vi "9_Meas_Tf.vi"(0 "file path (IN)":path, 1 "ICE":dbl, 5 "Project #":string, 7 "Request #":string, 9 "TEST #":string, 11 "error in (no error)":errorcluster) -> (4 "file path (OUT)":path, 6 "Tf (ns)":dbl, 8 "DONE Tf":bool, 10 "OFF Region":waveform(dbl)[](graph) caption="Tf (ns)", 15 "error out":errorcluster)   [LabVIEW 2020]
uses:
  <vilib>/Waveform/WDTOps.llb/WDT Waveform Duration DBL.vi
  <vilib>/Waveform/WDTOps.llb/WDT Get Waveform Subset DBL.vi
  <vilib>/measure/mascope.llb/Transition Measurements 1 chan.vi
  <vilib>/measure/NI_MAPro.lvlib
panel:
  in  "Decision ?":bool
  in  "Cursor b : Channel 1 \nfall edge tolerance":dbl=0.1
  in  "Cursor b : Channel 1 \nfall edge number":i32=1 min=1
  in  "Cursor a : Channel 1 \nfall edge tolerance":dbl=0.1
  in  "Cursor a : Channel 1 \nfall edge number":i32=1 min=1
  out "Cursor a : Channel 1":dbl
  out "Cursor b : Channel 1":dbl
  out "10% Ice":dbl
  out "90% Ice":dbl
  out "measurement info (CH1 Cursor a)":T1 {"ref levels"."ref units" items=["absolute", "relative"]; "ref levels"."high ref level" format="%.2p"; "ref levels"."low ref level" format="%.2p"; "ref levels"."mid ref level" format="%.2p"; "end time" format="%.6e"; "start time" format="%.6e"}
  out "measurement info (CH1 Cursor b)":T1 {"ref levels"."ref units" items=["absolute", "relative"]; "ref levels"."high ref level" format="%.2p"; "ref levels"."low ref level" format="%.2p"; "ref levels"."mid ref level" format="%.2p"; "end time" format="%.6e"; "start time" format="%.6e"}
  in  "reference  levels (CH1 2nd Cursor)":T2={"high ref level"=90.0, "mid ref level"=50.0, "low ref level"=10.0, "ref units"=1} {"ref units" items=["absolute", "percent"]; "high ref level" format="%0.2f"; "low ref level" format="%0.2f"; "mid ref level" format="%0.2f"}
  in  "reference  levels (CH1 1st Cursor)":T2={"high ref level"=90.0, "mid ref level"=50.0, "low ref level"=10.0, "ref units"=1} {"ref units" items=["absolute", "percent"]; "high ref level" format="%0.2f"; "low ref level" format="%0.2f"; "mid ref level" format="%0.2f"}
  out "Waveform Graph":waveform(dbl)[](graph)
  # "From 90% Ice to 10% Ice"
  # "Default = 1"
  # "Default = 1"
  # "Default = 0.1"
  # "Default = 0.1"
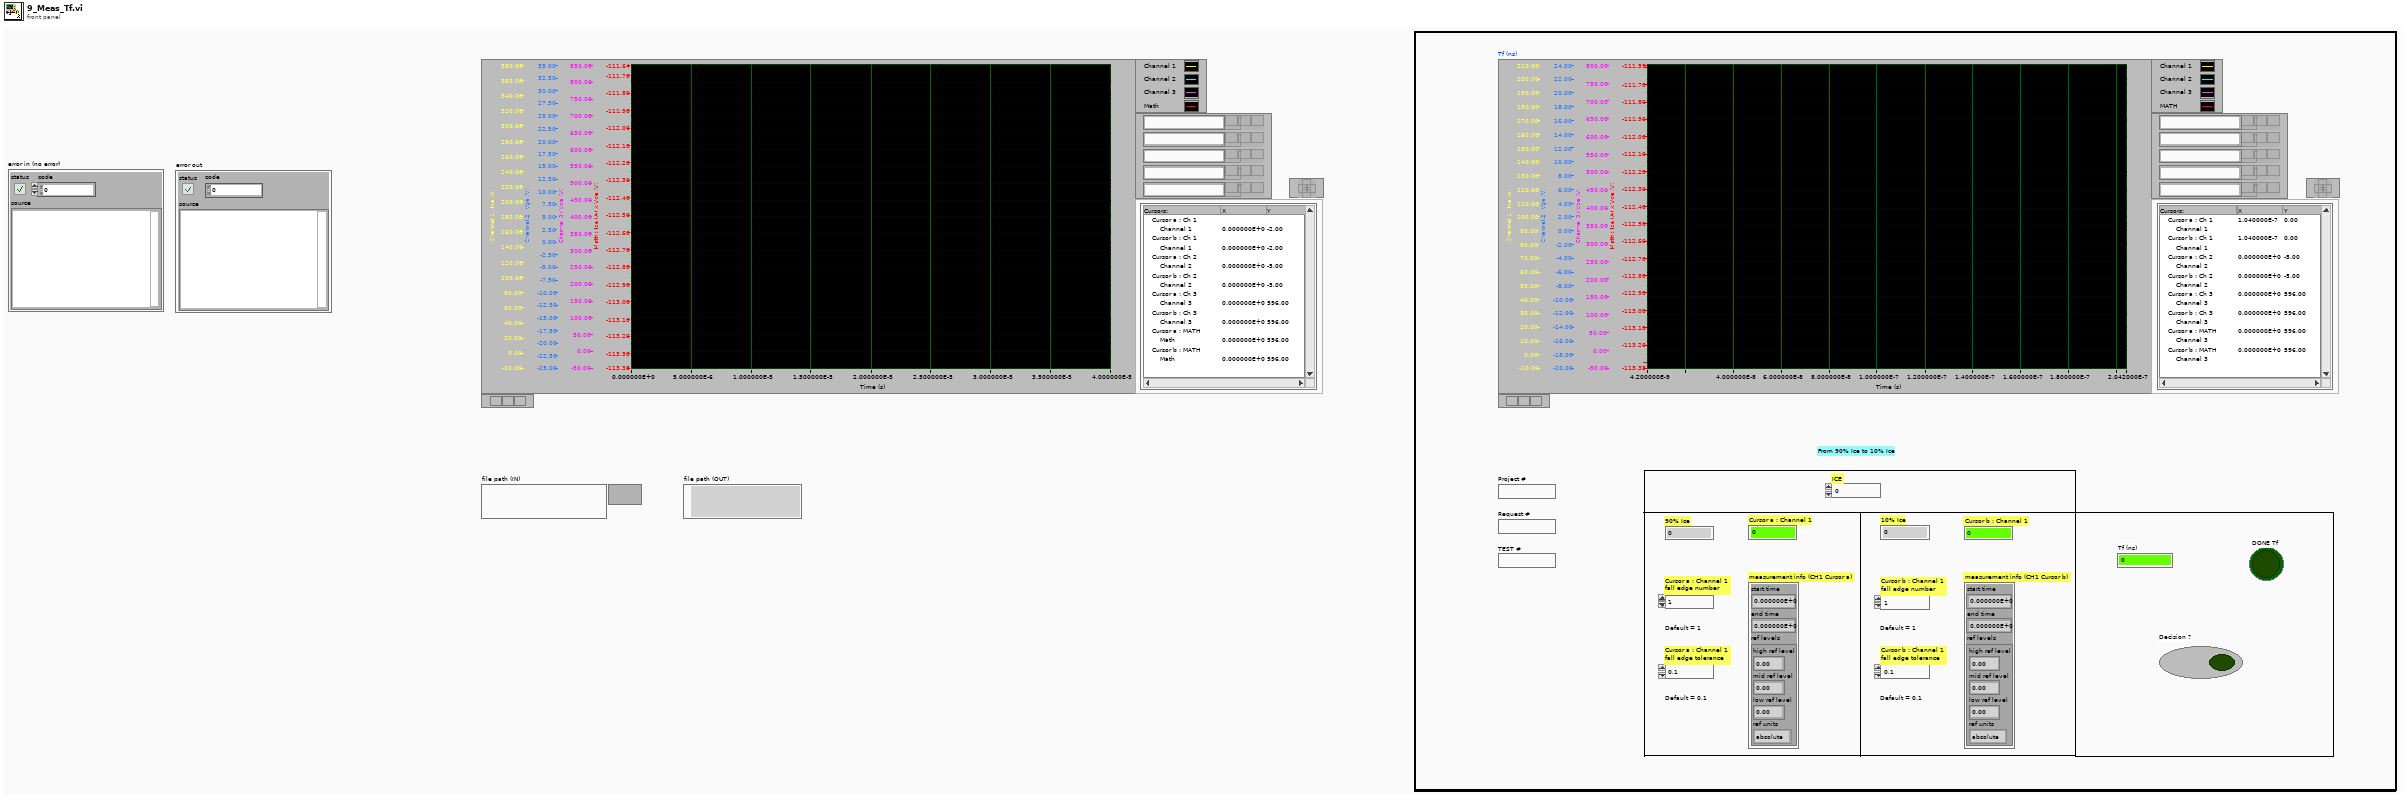
[diagram p1: front panel]
types:
  T1 = cluster{"start time":dbl, "end time":dbl, "ref levels":cluster{"high ref level":dbl, "mid ref level":dbl, "low ref level":dbl, "ref units":u16}}
  T2 = cluster{"high ref level":dbl, "mid ref level":dbl, "low ref level":dbl, "ref units":u16}
  T3 = enum32{"Invalid", "Standard", "Closed", "Hidden", "Minimized", "Maximized"}
  T4 = typedef "imagedata.ctl" = cluster{"image type":i32, "image depth":i32, "image":u8[], "mask":u8[], "colors":u32[], "Rectangle":cluster{"left":i16, "top":i16, "right":i16, "bottom":i16}}
diagram:
  w11 = 0.0 ("Cursor a : Channel 1")
  w13 = errorcluster {"status"=FALSE, "code"=0, "source"=""} ("error out")
  w12 = FALSE ("DONE Tdon")
  w14 = waveform(dbl)[] [] ("Waveform Graph")
  n1 = local write "Cursor a : Channel 1 \nfall edge tolerance"(0.1 ("Cursor a : Channel 1 \nfall edge tolerance")) -> ()
  n2 = local write "Cursor a : Channel 1 \nfall edge number"(1 ("Cursor a : Channel 1 \nfall edge number")) -> ()
  n3 = local write "Cursor b : Channel 1 \nfall edge tolerance"(0.1 ("Cursor b : Channel 1 \nfall edge tolerance")) -> ()
  n4 = local write "Cursor b : Channel 1 \nfall edge number"(1 ("Cursor b : Channel 1 \nfall edge number")) -> ()
  n5 = local write "error out"(w13) -> ()
  n6 = local write "error in (no error)"(w13) -> ()
  n7 = local write "Cursor a : Channel 1"(w11) -> ()
  n8 = local write "Cursor b : Channel 1"(w11) -> ()
  n9 = local write "DONE Tf"(w12) -> ()
  n10 = local write "Waveform Graph"(w14) -> ()
  n11 = local write "OFF Region"(w14) -> ()
  n12 = local write "Decision ?"(w12) -> ()
  n13 = local write "Tf (ns)"(w11) -> ()
  n14 = flat-sequence {
    tunnel: ["file path (IN)"] -> w6
    tunnel: [w15] -> w5
    tunnel: [w26] -> w10
    tunnel: [w25] -> w8
    tunnel: w6 -> [w24]
    tunnel: w5 -> [w23]
    tunnel: w10 -> [w247]
    tunnel: [w246] -> w9
    tunnel: w8 -> [w246]
    tunnel: [w245] -> w7
    tunnel: w9 -> [w261]
    tunnel: w7 -> [w260]
    frame #0 {
      n15 = control-ref of="This VI"() -> (w21:refnum<vi>)
      n16 = invoke class="VI" method="FP.Open"(reference=w21, error in="error in (no error)", "Activate"=TRUE ("Activate?"), "State"=T3."Maximized") -> (error out=w22:errorcluster)  [unwired: 1 in, 4 out]
      n17 = property class="VI"(reference=w21, error in=w22, "Front Panel.Closeable"=TRUE ("Front Panel Window:Closeable")) -> (error out=w15:errorcluster)  [unwired: 1 out]
    }
    frame #1 {
      n18 = while {
        shift-right: [w32] -> w26
        shift-left: w23 -> [w31]
        tunnel: [w28] -> w25
        tunnel: w24 -> [w27]
        stop <- w33 stop-if-true
        n19 = flat-sequence {
          tunnel: w31 -> [w62]
          tunnel: [w62] -> w30
          tunnel: [w57] -> w29
          tunnel: w27 -> [w57]
          tunnel: [w78] -> w50
          tunnel: [w77] -> w49
          tunnel: [w67] -> w48
          tunnel: w30 -> [w155]
          tunnel: w29 -> [w149]
          tunnel: w50 -> [w184]
          tunnel: w49 -> [w198]
          tunnel: [w178] -> w47
          tunnel: w48 -> [w191]
          tunnel: [w191] -> w46
          tunnel: [w177] -> w45
          tunnel: [w176] -> w44
          tunnel: [w175] -> w43
          tunnel: [w174] -> w42
          tunnel: w47 -> [w226]
          tunnel: [w225] -> w41
          tunnel: w46 -> [w227]
          tunnel: [w227] -> w40
          tunnel: w45 -> [_]
          tunnel: w44 -> [_]
          tunnel: w43 -> [w219]
          tunnel: [w219] -> w39
          tunnel: w42 -> [w220]
          tunnel: [w220] -> w38
          tunnel: w41 -> [w228]
          tunnel: w40 -> [w234]
          tunnel: [w234] -> w37
          tunnel: w39 -> [w232]
          tunnel: w38 -> [w231]
          tunnel: [w228] -> w36
          tunnel: w37 -> [w239]
          tunnel: w36 -> [w241]
          tunnel: [w240] -> w35
          tunnel: [w239] -> w28
          frame #0 {
            w60 = 0.0 ("Cursor a : Channel 1")
            w59 = FALSE ("DONE Tdon")
            w58 = waveform(dbl)[] [] ("Waveform Graph")
            n20 = Wait (ms)(milliseconds to wait=u32 200) -> ()  [unwired: 1 out]
            n21 = local write "Cursor a : Channel 1"(w60) -> ()
            n22 = local write "Cursor b : Channel 1"(w60) -> ()
            n23 = local write "DONE Tf"(w59) -> ()
            n24 = local write "Waveform Graph"(w58) -> ()
            n25 = local write "OFF Region"(w58) -> ()
            n26 = local write "Decision ?"(w59) -> ()
            n27 = local write "Tf (ns)"(w60) -> ()
          }
          frame #1 {
            w63 = 0.0 ("start samples/time")
            w130 = u16 1 items=["Samples", "Relative Time"] ("start/duration format")
            w141 = u16 1 items=["Samples", "Relative Time"] ("start/duration format")
            w142 = u16 1 items=["Samples", "Relative Time"] ("start/duration format")
            # "Channel 1"
            # "Channel 3"
            # "Channel 2"
            # "dt"
            # "Ch2"
            # "Ch1"
            n28 = call "3_ReadDatatoWaveform.vi"("error in (no error)"=w155, "file path (IN)"=w149) -> ("error out"=w123:errorcluster, "Waveform Graph"=→"Waveform Graph":waveform(dbl)[], "file path (OUT)"=w67:path, "dt"=w150:dbl, "Ch 2 Data"=w147:dbl[], "Ch 3 Data"=w151:dbl[], "Ch 1 Data"=w148:dbl[])  [unwired: 3 in]
            n29 = To Time Stamp(1:0.0 ("number")) -> (0:w152:timestamp)
            n30 = disable-structure shown="Enabled" {
              disable-tunnel: w152 -> [w159 _]
              disable-tunnel: w150 -> [w158 _]
              disable-tunnel: w148 -> [w157 _]
              disable-tunnel: [w156 _] -> w129
              frame Enabled {
                # "Channel 1"
                n31 = Bundle By Name("Y"=w157, "dt"=w158, "t0"=w159) -> (w156:waveform(dbl))  [unwired: 1 in]
              }
              frame Disabled {
              }
            }
            n32 = disable-structure shown="Enabled" {
              disable-tunnel: w152 -> [w163 _]
              disable-tunnel: w150 -> [w162 _]
              disable-tunnel: w147 -> [w161 _]
              disable-tunnel: [w160 _] -> w128
              frame Enabled {
                # "Channel 2"
                n33 = Bundle By Name("Y"=w161, "dt"=w162, "t0"=w163) -> (w160:waveform(dbl))  [unwired: 1 in]
              }
              frame Disabled {
              }
            }
            n34 = disable-structure shown="Enabled" {
              disable-tunnel: w152 -> [w167 _]
              disable-tunnel: w150 -> [w166 _]
              disable-tunnel: w151 -> [w165 _]
              disable-tunnel: [w164 _] -> w127
              frame Enabled {
                # "Channel 3"
                n35 = Bundle By Name("Y"=w165, "dt"=w166, "t0"=w167) -> (w164:waveform(dbl))  [unwired: 1 in]
              }
              frame Disabled {
              }
            }
            n36 = call-poly <vilib>:"Waveform Duration.vi"("error in (no error)"=w123, "waveform in"=w127) -> ("error out"=w135:errorcluster, "duration"=w132:dbl, "waveform out"=w134:waveform(dbl))  [unwired: 7 in]
            n37 = call-poly <vilib>:"Waveform Duration.vi"("error in (no error)"=w123, "waveform in"=w128) -> ("error out"=w136:errorcluster, "duration"=w139:dbl, "waveform out"=w137:waveform(dbl))  [unwired: 7 in]
            n38 = call-poly <vilib>:"Waveform Duration.vi"("error in (no error)"=w123, "waveform in"=w129) -> ("error out"=w146:errorcluster, "duration"=w143:dbl, "waveform out"=w145:waveform(dbl))  [unwired: 7 in]
            n39 = Divide(x=w132, y=2.0) -> (x/y=w131:dbl)
            n40 = Divide(x=w139, y=2.0) -> (x/y=w140:dbl)
            n41 = Divide(x=w143, y=2.0) -> (x/y=w124:dbl)
            n42 = call-poly <vilib>:"Get Waveform Subset.vi"("start/duration format"=w130, "error in (no error)"=w135, "duration"=w131, "start samples/time"=w63, "waveform in"=w134) -> ("error out"=w120:errorcluster, "waveform out"=w126:waveform(dbl))  [unwired: 1 in, 2 out]
            n43 = call-poly <vilib>:"Get Waveform Subset.vi"("start/duration format"=w141, "error in (no error)"=w136, "duration"=w140, "start samples/time"=w63, "waveform in"=w137) -> ("error out"=w121:errorcluster, "waveform out"=w79:waveform(dbl))  [unwired: 1 in, 2 out]
            n44 = call-poly <vilib>:"Get Waveform Subset.vi"("start/duration format"=w142, "error in (no error)"=w146, "duration"=w124, "start samples/time"=w63, "waveform in"=w145) -> ("error out"=w122:errorcluster, "waveform out"=w78:waveform(dbl))  [unwired: 1 in, 2 out]
            n45 = Build Array(w78, w79, w126) -> (→"OFF Region":waveform(dbl)[])
            n46 = Merge Errors(w122, w121, w120) -> (w75:errorcluster)
            n47 = property on="OFF Region" class="WFGraph (strict)"(error in=w75) -> (error out=w74:errorcluster, "Width"=w73:u32)  [unwired: 1 in, 1 out]
            n48 = property on="OFF Region" class="WFGraph (strict)"(error in=w74, "Caption.Justify"=enum16{"Left", "Center", "Right"}."Left" ("Caption.Justification"), "Caption.Width"=w73, "Caption.FontBold"=TRUE ("Caption.Font:Bold"), "Caption.FontColor"=u32 16860 ("Caption.Font:Color"), "Caption.FontSize"=u32 24 ("Caption.Font:Size"), "Caption.Text"="Tf (ns)") -> (error out=w69:errorcluster)  [unwired: 1 in, 1 out]
            n49 = property on="OFF Region" class="WFGraph (strict)"(error in=w69, "XScale.Offset"=w63) -> (error out=w103:errorcluster)  [unwired: 1 in, 1 out]
            n50 = property on="OFF Region" class="WFGraph (strict)"(error in=w103, "Active Cursor"=u32 0, "Cursor.Cursor X"=0.0 ("Cursor.Cursor Position:Cursor X"), "Cursor.Cursor Y"=0.0 ("Cursor.Cursor Position:Cursor Y"), "Cursor.Visible"=FALSE) -> (error out=w102:errorcluster)  [unwired: 1 in, 1 out]
            n51 = property on="OFF Region" class="WFGraph (strict)"(error in=w102, "Active Cursor"=u32 1, "Cursor.Cursor X"=0.0 ("Cursor.Cursor Position:Cursor X"), "Cursor.Cursor Y"=0.0 ("Cursor.Cursor Position:Cursor Y"), "Cursor.Visible"=FALSE) -> (error out=w101:errorcluster)  [unwired: 1 in, 1 out]
            n52 = property on="OFF Region" class="WFGraph (strict)"(error in=w101, "Active Cursor"=u32 2, "Cursor.Cursor X"=0.0 ("Cursor.Cursor Position:Cursor X"), "Cursor.Cursor Y"=0.0 ("Cursor.Cursor Position:Cursor Y"), "Cursor.Visible"=FALSE) -> (error out=w100:errorcluster)  [unwired: 1 in, 1 out]
            n53 = property on="OFF Region" class="WFGraph (strict)"(error in=w100, "Active Cursor"=u32 3, "Cursor.Cursor X"=0.0 ("Cursor.Cursor Position:Cursor X"), "Cursor.Cursor Y"=0.0 ("Cursor.Cursor Position:Cursor Y"), "Cursor.Visible"=FALSE) -> (error out=w83:errorcluster)  [unwired: 1 in, 1 out]
            n54 = property on="OFF Region" class="WFGraph (strict)"(error in=w83, "Active Cursor"=u32 4, "Cursor.Cursor X"=0.0 ("Cursor.Cursor Position:Cursor X"), "Cursor.Cursor Y"=0.0 ("Cursor.Cursor Position:Cursor Y"), "Cursor.Visible"=FALSE) -> (error out=w82:errorcluster)  [unwired: 1 in, 1 out]
            n55 = property on="OFF Region" class="WFGraph (strict)"(error in=w82, "Active Cursor"=u32 5, "Cursor.Cursor X"=0.0 ("Cursor.Cursor Position:Cursor X"), "Cursor.Cursor Y"=0.0 ("Cursor.Cursor Position:Cursor Y"), "Cursor.Visible"=FALSE) -> (error out=w81:errorcluster)  [unwired: 1 in, 1 out]
            n56 = property on="OFF Region" class="WFGraph (strict)"(error in=w81, "Active Cursor"=u32 6, "Cursor.Cursor X"=0.0 ("Cursor.Cursor Position:Cursor X"), "Cursor.Cursor Y"=0.0 ("Cursor.Cursor Position:Cursor Y"), "Cursor.Visible"=FALSE) -> (error out=w80:errorcluster)  [unwired: 1 in, 1 out]
            n57 = property on="OFF Region" class="WFGraph (strict)"(error in=w80, "Active Cursor"=u32 7, "Cursor.Cursor X"=0.0 ("Cursor.Cursor Position:Cursor X"), "Cursor.Cursor Y"=0.0 ("Cursor.Cursor Position:Cursor Y"), "Cursor.Visible"=FALSE) -> (error out=w77:errorcluster)  [unwired: 1 in, 1 out]
            n58 = call <vilib>:"Beep.vi"("use system alert? (T)"=FALSE, "duration (msec)"=u32 200, "frequency (Hz)"=u32 2000) -> ()  [unwired: 9 in]
          }
          frame #2 {
            w211 = u16 0 items=["falling", "rising"] ("polarity (rising)")
            w212 = u16 0 items=["falling", "rising"] ("polarity (rising)")
            # "Cursor a : Channel 1"
            # "Cursor b : Channel 1"
            # "Cursor b : Channel 1"
            # "Cursor a : Channel 1"
            # "Cursor b : Channel 1"
            # "Cursor a : Channel 1"
            # "Cursor b : Channel 1"
            # "Cursor a : Channel 1"
            # "End Time 1st Cursor"
            # "End Time 2nd Cursor"
            # "1st PARAMETER : 90% Ice"
            # "Channel 1"
            # "2nd PARAMETER : 10% Ice"
            # "Channel 1"
            n59 = Divide(x=90.0, y=100.0) -> (x/y=w218:dbl)
            n60 = Multiply(x=w218, y="ICE") -> (x*y=w186:dbl)
            "90% Ice" <- w186
            n61 = Add(x=w186, y="Cursor a : Channel 1 \nfall edge tolerance") -> (x+y=w204:dbl)
            n62 = Subtract(x=w186, y="Cursor a : Channel 1 \nfall edge tolerance") -> (x-y=w203:dbl)
            n63 = Bundle By Name(cluster="reference  levels (CH1 1st Cursor)", "high ref level"=w204, "mid ref level"=w186, "low ref level"=w203, "ref units"=u16 0) -> (w200:T2)
            n64 = call-poly <vilib>:"Transition Measurements.vi"("edge number (1)"="Cursor a : Channel 1 \nfall edge number", "error in (no error)"=w198, "reference levels"=w200, "polarity (rising)"=w212, "signal in"=w184) -> ("error out"=w195:errorcluster, "measurement info"=w199:T1)  [unwired: 1 in, 4 out]
            "measurement info (CH1 Cursor a)" <- w199
            n65 = Unbundle By Name(w199) -> ("end time"=w174:dbl)
            n66 = property on="OFF Region" class="WFGraph (strict)"(error in=w195, "Active Cursor"=u32 0, "Cursor.Cursor X"=w174, "Cursor.Visible"=TRUE, "Cursor.Cursor Name Visible"=TRUE) -> (error out=w183:errorcluster)  [unwired: 1 in, 1 out]
            n67 = property on="OFF Region" class="WFGraph (strict)"(error in=w183, "Active Cursor"=u32 0) -> (error out=w181:errorcluster, "Cursor.Cursor Y"=w177:dbl)  [unwired: 1 in, 1 out]
            "Cursor a : Channel 1" <- w177
            n68 = Divide(x=10.0, y=100.0) -> (x/y=w215:dbl)
            n69 = Multiply(x=w215, y="ICE") -> (x*y=w187:dbl)
            "10% Ice" <- w187
            n70 = Add(x=w187, y="Cursor b : Channel 1 \nfall edge tolerance") -> (x+y=w210:dbl)
            n71 = Subtract(x=w187, y="Cursor b : Channel 1 \nfall edge tolerance") -> (x-y=w209:dbl)
            n72 = Bundle By Name(cluster="reference  levels (CH1 2nd Cursor)", "high ref level"=w210, "mid ref level"=w187, "low ref level"=w209, "ref units"=u16 0) -> (w206:T2)
            n73 = call-poly <vilib>:"Transition Measurements.vi"("edge number (1)"="Cursor b : Channel 1 \nfall edge number", "error in (no error)"=w181, "reference levels"=w206, "polarity (rising)"=w211, "signal in"=w184) -> ("error out"=w192:errorcluster, "measurement info"=w205:T1)  [unwired: 1 in, 4 out]
            "measurement info (CH1 Cursor b)" <- w205
            n74 = Unbundle By Name(w205) -> ("end time"=w175:dbl)
            n75 = property on="OFF Region" class="WFGraph (strict)"(error in=w192, "Active Cursor"=u32 1, "Cursor.Cursor X"=w175, "Cursor.Visible"=TRUE, "Cursor.Cursor Name Visible"=TRUE) -> (error out=w179:errorcluster)  [unwired: 1 in, 1 out]
            n76 = call <vilib>:"Beep.vi"("use system alert? (T)"=FALSE, "duration (msec)"=u32 200, "frequency (Hz)"=u32 2000) -> ()  [unwired: 9 in]
            n77 = property on="OFF Region" class="WFGraph (strict)"(error in=w179, "Active Cursor"=u32 1) -> (error out=w178:errorcluster, "Cursor.Cursor Y"=w176:dbl)  [unwired: 1 in, 1 out]
            "Cursor b : Channel 1" <- w176
          }
          frame #3 {
            # "2nd Cursor"
            # "1st Cursor"
            n78 = Subtract(x=w220, y=1e-07) -> (x-y=w221:dbl)
            n79 = Add(x=w219, y=1e-07) -> (x+y=w222:dbl)
            n80 = property on="OFF Region" class="WFGraph (strict)"(error in=w226, "XScale.Minimum"=w221, "XScale.Maximum"=w222) -> (error out=w225:errorcluster)  [unwired: 1 in, 1 out]
          }
          frame #4 {
            # "ns"
            n81 = Subtract(x=w232, y=w231) -> (x-y=w230:dbl)
            n82 = Absolute Value(x=w230) -> (abs(x)=w229:dbl)
            n83 = Multiply(x=w229, y=1000000000.0) -> (x*y=→"Tf (ns)":dbl)
            n84 = call <vilib>:"Beep.vi"("use system alert? (T)"=FALSE, "duration (msec)"=u32 200, "frequency (Hz)"=u32 2000) -> ()  [unwired: 9 in]
          }
          frame #5 {
            n85 = while {
              shift-right: [w242] -> w240
              shift-left: w241 -> [w242]
              stop <- "Decision ?" stop-if-true
              n86 = Wait (ms)(milliseconds to wait=u32 100) -> ()  [unwired: 1 out]
            }
          }
        }
        n87 = while {
          tunnel: [w52] -> w33
          shift-right: [w55] -> w32
          shift-left: w35 -> [w56]
          stop <- w54 stop-if-true
          n88 = Wait (ms)(milliseconds to wait=u32 100) -> ()  [unwired: 1 out]
          n89 = call "Display Message to User"("error in (no error)"=w56) -> ("error out"=w55:errorcluster, "NO"=w52:bool)  [unwired: 9 in]
          n90 = Or(x=w52, y=TRUE) -> (x .or. y?=w54:bool)
        }
        n91 = Wait (ms)(milliseconds to wait=u32 100) -> ()  [unwired: 1 out]
      }
    }
    frame #2 {
      w251 = "_"
      n92 = invoke on="OFF Region" class="WFGraph (strict)" method="Get Image"(error in=w247) -> (error out=w253:errorcluster, "image data"=w256:T4)  [unwired: 5 in, 4 out]
      n93 = Concatenate Strings("C:\\Inductive_Switching_Project\\IndSw_Image\\" ("string"), "Project #", w251, "Request #", w251, "TEST #", w251, "Tf" ("string"), ".png" ("string")) -> (w257:string)
      n94 = String To Path(string=w257) -> (path=w255:path)
      n95 = call <vilib>:"Write PNG File.vi"("error in (no error)"=w253, "image data"=w256, "path to PNG file"=w255) -> ("error out"=w245:errorcluster)  [unwired: 7 in, 1 out]
      "DONE Tf" <- TRUE ("DONE Tdon")
    }
    frame #3 {
      n96 = disable-structure shown="Enabled" {
        disable-tunnel: w260 -> [w262 _]
        frame Enabled {
          n97 = control-ref of="This VI"() -> (w263:refnum<vi>)
          n98 = invoke class="VI" method="FP.Close"(reference=w263, error in=w262) -> ()  [unwired: 1 in, 3 out]
        }
        frame Disabled {
        }
      }
      "error out" <- w260
      "file path (OUT)" <- w261
    }
  }
